vi "rszvl_core_global.vi"() -> ()   [LabVIEW 2014] (continued)
{"Name"="rszvl_rngTrigMode", "Type"=2, "Min?"=FALSE, "Max?"=FALSE, "Entries"=[{"Name"="RSZVL_VAL_TRIG_MODE_IMM", "Discrete or Min"=0.0, "Max"=0.0, "Coerced"=0.0, "Command"="IMM"}, {"Name"="RSZVL_VAL_TRIG_MODE_EXT", "Discrete or Min"=1.0, "Max"=0.0, "Coerced"=0.0, "Command"="EXT"}, {"Name"="RSZVL_VAL_TRIG_MODE_POW", "Discrete or Min"=2.0, "Max"=0.0, "Coerced"=0.0, "Command"="POW"}]}, {"Name"="rszvl_rngWlanDemod", "Type"=2, "Min?"=FALSE, "Max?"=FALSE, "Entries"=[{"Name"="RSZVL_VAL_WLAN_BPSK", "Discrete or Min"=0.0, "Max"=0.0, "Coerced"=0.0, "Command"="BPSK"}, {"Name"="RSZVL_VAL_WLAN_QPSK", "Discrete or Min"=1.0, "Max"=0.0, "Coerced"=0.0, "Command"="QPSK"}, {"Name"="RSZVL_VAL_WLAN_QAM16", "Discrete or Min"=2.0, "Max"=0.0, "Coerced"=0.0, "Command"="QAM16"}, {"Name"="RSZVL_VAL_WLAN_QAM64", "Discrete or Min"=3.0, "Max"=0.0, "Coerced"=0.0, "Command"="QAM64"}, {"Name"="RSZVL_VAL_WLAN_BPSK6", "Discrete or Min"=4.0, "Max"=0.0, "Coerced"=0.0, "Command"="BPSK6"}, {"Name"="RSZVL_VAL_WLAN_BPSK9", "Discrete or Min"=5.0, "Max"=0.0, "Coerced"=0.0, "Command"="BPSK9"}, {"Name"="RSZVL_VAL_WLAN_QPSK12", "Discrete or Min"=6.0, "Max"=0.0, "Coerced"=0.0, "Command"="QPSK12"}, {"Name"="RSZVL_VAL_WLAN_QPSK18", "Discrete or Min"=7.0, "Max"=0.0, "Coerced"=0.0, "Command"="QPSK18"}, {"Name"="RSZVL_VAL_WLAN_QAM1624", "Discrete or Min"=8.0, "Max"=0.0, "Coerced"=0.0, "Command"="QAM1624"}, {"Name"="RSZVL_VAL_WLAN_QAM1636", "Discrete or Min"=9.0, "Max"=0.0, "Coerced"=0.0, "Command"="QAM1636"}, {"Name"="RSZVL_VAL_WLAN_QAM6448", "Discrete or Min"=10.0, "Max"=0.0, "Coerced"=0.0, "Command"="QAM6448"}, {"Name"="RSZVL_VAL_WLAN_QAM6454", "Discrete or Min"=11.0, "Max"=0.0, "Coerced"=0.0, "Command"="QAM6454"}, {"Name"="RSZVL_VAL_WLAN_DBPSK", "Discrete or Min"=12.0, "Max"=0.0, "Coerced"=0.0, "Command"="DBPSK1"}, {"Name"="RSZVL_VAL_WLAN_DQPSK", "Discrete or Min"=13.0, "Max"=0.0, "Coerced"=0.0, "Command"="DQPSK2"}, {"Name"="RSZVL_VAL_WLAN_CCK55", "Discrete or Min"=14.0, "Max"=0.0, "Coerced"=0.0, "Command"="CCK55"}, {"Name"="RSZVL_VAL_WLAN_CCK11", "Discrete or Min"=15.0, "Max"=0.0, "Coerced"=0.0, "Command"="CCK11"}, {"Name"="RSZVL_VAL_WLAN_PBCC55", "Discrete or Min"=16.0, "Max"=0.0, "Coerced"=0.0, "Command"="PBCC55"}, {"Name"="RSZVL_VAL_WLAN_PBCC11", "Discrete or Min"=17.0, "Max"=0.0, "Coerced"=0.0, "Command"="PBCC11"}, {"Name"="RSZVL_VAL_WLAN_PBCC22", "Discrete or Min"=18.0, "Max"=0.0, "Coerced"=0.0, "Command"="PBCC22"}, {"Name"="RSZVL_VAL_WLAN_BPSK3", "Discrete or Min"=19.0, "Max"=0.0, "Coerced"=0.0, "Command"="BPSK3"}, {"Name"="RSZVL_VAL_WLAN_BPSK45", "Discrete or Min"=20.0, "Max"=0.0, "Coerced"=0.0, "Command"="BPSK45"}, {"Name"="RSZVL_VAL_WLAN_QPSK6", "Discrete or Min"=21.0, "Max"=0.0, "Coerced"=0.0, "Command"="QPSK6"}, {"Name"="RSZVL_VAL_WLAN_QPSK9", "Discrete or Min"=22.0, "Max"=0.0, "Coerced"=0.0, "Command"="QPSK9"}, {"Name"="RSZVL_VAL_WLAN_QAM1612", "Discrete or Min"=23.0, "Max"=0.0, "Coerced"=0.0, "Command"="QAM1612"}, {"Name"="RSZVL_VAL_WLAN_QAM1618", "Discrete or Min"=24.0, "Max"=0.0, "Coerced"=0.0, "Command"="QAM1618"}, {"Name"="RSZVL_VAL_WLAN_QAM6424", "Discrete or Min"=25.0, "Max"=0.0, "Coerced"=0.0, "Command"="QAM6424"}, {"Name"="RSZVL_VAL_WLAN_QAM6427", "Discrete or Min"=26.0, "Max"=0.0, "Coerced"=0.0, "Command"="QAM6427"}]}, {"Name"="rszvl_rngWlanDbyte", "Type"=0, "Min?"=TRUE, "Max?"=TRUE, "Entries"=[{"Name"="", "Discrete or Min"=1.0, "Max"=4095.0, "Coerced"=0.0, "Command"=""}]}, {"Name"="rszvl_rngWiMaxStandard", "Type"=0, "Min?"=TRUE, "Max?"=TRUE, "Entries"=[{"Name"="", "Discrete or Min"=0.0, "Max"=2.0, "Coerced"=0.0, "Command"=""}]}, {"Name"="rszvl_rngWiMAXFreqBand", "Type"=2, "Min?"=FALSE, "Max?"=FALSE, "Entries"=[{"Name"="RSZVL_VAL_WIMAX_FBAN_UNSP", "Discrete or Min"=0.0, "Max"=0.0, "Coerced"=0.0, "Command"="UNSP"}, {"Name"="RSZVL_VAL_WIMAX_FBAN_ETSI", "Discrete or Min"=1.0, "Max"=0.0, "Coerced"=0.0, "Command"="ETSI"}, {"Name"="RSZVL_VAL_WIMAX_FBAN_MMDS", "Discrete or Min"=2.0, "Max"=0.0, "Coerced"=0.0, "Command"="MMDS"}, {"Name"="RSZVL_VAL_WIMAX_FBAN_WCS", "Discrete or Min"=3.0, "Max"=0.0, "Coerced"=0.0, "Command"="WCS"}, {"Name"="RSZVL_VAL_WIMAX_FBAN_CEPT", "Discrete or Min"=4.0, "Max"=0.0, "Coerced"=0.0, "Command"="CEPT"}, {"Name"="RSZVL_VAL_WIMAX_FBAN_UNI", "Discrete or Min"=5.0, "Max"=0.0, "Coerced"=0.0, "Command"="UNII"}, {"Name"="RSZVL_VAL_WIMAX_FBAN_ETSI2", "Discrete or Min"=6.0, "Max"=0.0, "Coerced"=0.0, "Command"="ETSI2"}, {"Name"="RSZVL_VAL_WIMAX_FBAN_MMDS2", "Discrete or Min"=7.0, "Max"=0.0, "Coerced"=0.0, "Command"="MMDS2"}, {"Name"="RSZVL_VAL_WIMAX_FBAN_WCS2", "Discrete or Min"=8.0, "Max"=0.0, "Coerced"=0.0, "Command"="WCS2"}, {"Name"="RSZVL_VAL_WIMAX_FBAN_CEPT2", "Discrete or Min"=9.0, "Max"=0.0, "Coerced"=0.0, "Command"="CEPT2"}, {"Name"="RSZVL_VAL_WIMAX_FBAN_UNI2", "Discrete or Min"=10.0, "Max"=0.0, "Coerced"=0.0, "Command"="UNII2"}]}, {"Name"="rszvl_rngWiMAXGuardRatio", "Type"=1, "Min?"=FALSE, "Max?"=FALSE, "Entries"=[{"Name"="", "Discrete or Min"=0.0, "Max"=0.0, "Coerced"=4.0, "Command"=""}, {"Name"="", "Discrete or Min"=0.0, "Max"=0.0, "Coerced"=8.0, "Command"=""}, {"Name"="", "Discrete or Min"=0.0, "Max"=0.0, "Coerced"=16.0, "Command"=""}, {"Name"="", "Discrete or Min"=0.0, "Max"=0.0, "Coerced"=32.0, "Command"=""}]}, {"Name"="rszvl_rngWiMAXRSSIAver", "Type"=0, "Min?"=TRUE, "Max?"=TRUE, "Entries"=[{"Name"="", "Discrete or Min"=1e-06, "Max"=0.999999, "Coerced"=0.0, "Command"=""}]}, {"Name"="rszvl_rngWiMAXModulForm", "Type"=2, "Min?"=FALSE, "Max?"=FALSE, "Entries"=[{"Name"="RSZVL_VAL_WIMAX_MODUL_ALL", "Discrete or Min"=0.0, "Max"=0.0, "Coerced"=0.0, "Command"="ALL"}, {"Name"="RSZVL_VAL_WIMAX_MODUL_QPSK", "Discrete or Min"=1.0, "Max"=0.0, "Coerced"=0.0, "Command"="QPSK"}, {"Name"="RSZVL_VAL_WIMAX_MODUL_QAM16", "Discrete or Min"=2.0, "Max"=0.0, "Coerced"=0.0, "Command"="QAM16"}, {"Name"="RSZVL_VAL_WIMAX_MODUL_QAM64", "Discrete or Min"=3.0, "Max"=0.0, "Coerced"=0.0, "Command"="QAM64"}, {"Name"="RSZVL_VAL_WIMAX_MODUL_BPSK", "Discrete or Min"=4.0, "Max"=0.0, "Coerced"=0.0, "Command"="BPSK"}]}, {"Name"="rszvl_rngWiMAXBurstNumber", "Type"=0, "Min?"=TRUE, "Max?"=TRUE, "Entries"=[{"Name"="", "Discrete or Min"=0.0, "Max"=9999.0, "Coerced"=0.0, "Command"=""}]}, {"Name"="rszvl_rngWiMAXPvtSel", "Type"=2, "Min?"=FALSE, "Max?"=FALSE, "Entries"=[{"Name"="RSZVL_VAL_PVT_EDGE", "Discrete or Min"=0.0, "Max"=0.0, "Coerced"=0.0, "Command"="EDGE"}, {"Name"="RSZVL_VAL_PVT_FULL", "Discrete or Min"=1.0, "Max"=0.0, "Coerced"=0.0, "Command"="FULL"}]}, {"Name"="rszvl_rngHzDeg", "Type"=2, "Min?"=FALSE, "Max?"=FALSE, "Entries"=[{"Name"="RSZVL_VAL_UNIT_DEG", "Discrete or Min"=9.0, "Max"=0.0, "Coerced"=0.0, "Command"="DEG"}, {"Name"="RSZVL_VAL_UNIT_HZ", "Discrete or Min"=12.0, "Max"=0.0, "Coerced"=0.0, "Command"="HZ"}]}, {"Name"="rszvl_rngWiMAXAcpChanNum", "Type"=0, "Min?"=TRUE, "Max?"=TRUE, "Entries"=[{"Name"="", "Discrete or Min"=0.0, "Max"=12.0, "Coerced"=0.0, "Command"=""}]}, {"Name"="rszvl_rngWiMAXChannelBw", "Type"=0, "Min?"=TRUE, "Max?"=TRUE, "Entries"=[{"Name"="", "Discrete or Min"=0.0, "Max"=100000000000.0, "Coerced"=0.0, "Command"=""}]}, {"Name"="rszvl_rngWiMAXChannelSpacing", "Type"=0, "Min?"=TRUE, "Max?"=TRUE, "Entries"=[{"Name"="", "Discrete or Min"=0.0, "Max"=100000000000.0, "Coerced"=0.0, "Command"=""}]}, {"Name"="rszvl_rngWiMAXFlatSel", "Type"=2, "Min?"=FALSE, "Max?"=FALSE, "Entries"=[{"Name"="RSZVL_VAL_WIMAX_FLAT_FLAT", "Discrete or Min"=0.0, "Max"=0.0, "Coerced"=0.0, "Command"="FLAT"}, {"Name"="RSZVL_VAL_WIMAX_FLAT_GRD", "Discrete or Min"=1.0, "Max"=0.0, "Coerced"=0.0, "Command"="GRD"}, {"Name"="RSZVL_VAL_WIMAX_FLAT_DIF", "Discrete or Min"=2.0, "Max"=0.0, "Coerced"=0.0, "Command"="DIFF"}]}, {"Name"="rszvl_rngWiMAXACPRSweepTime", "Type"=0, "Min?"=TRUE, "Max?"=TRUE, "Entries"=[{"Name"="", "Discrete or Min"=0.015, "Max"=16000.0, "Coerced"=0.0, "Command"=""}]}, {"Name"="rszvl_rngWiMAXDemod", "Type"=2, "Min?"=FALSE, "Max?"=FALSE, "Entries"=[{"Name"="RSZVL_VAL_WIMAX_BPSK1_2", "Discrete or Min"=0.0, "Max"=0.0, "Coerced"=0.0, "Command"="BPSK1/2"}, {"Name"="RSZVL_VAL_WIMAX_QPSK1_2", "Discrete or Min"=1.0, "Max"=0.0, "Coerced"=0.0, "Command"="QPSK1/2"}, {"Name"="RSZVL_VAL_WIMAX_QPSK3_4", "Discrete or Min"=2.0, "Max"=0.0, "Coerced"=0.0, "Command"="QPSK3/4"}, {"Name"="RSZVL_VAL_WIMAX_16QAM1_2", "Discrete or Min"=3.0, "Max"=0.0, "Coerced"=0.0, "Command"="16QAM1/2"}, {"Name"="RSZVL_VAL_WIMAX_16QAM3_4", "Discrete or Min"=4.0, "Max"=0.0, "Coerced"=0.0, "Command"="16QAM3/4"}, {"Name"="RSZVL_VAL_WIMAX_64QAM2_3", "Discrete or Min"=5.0, "Max"=0.0, "Coerced"=0.0, "Command"="64QAM2/3"}, {"Name"="RSZVL_VAL_WIMAX_64QAM3_4", "Discrete or Min"=6.0, "Max"=0.0, "Coerced"=0.0, "Command"="64QAM3/4"}]}, {"Name"="rszvl_rngWiMAXBconAuto", "Type"=2, "Min?"=FALSE, "Max?"=FALSE, "Entries"=[{"Name"="RSZVL_VAL_WIMAX_BCON_NONE", "Discrete or Min"=0.0, "Max"=0.0, "Coerced"=0.0, "Command"="NONE"}, {"Name"="RSZVL_VAL_WIMAX_BCON_FIRST", "Discrete or Min"=1.0, "Max"=0.0, "Coerced"=0.0, "Command"="FIRS"}, {"Name"="RSZVL_VAL_WIMAX_BCON_USER", "Discrete or Min"=2.0, "Max"=0.0, "Coerced"=0.0, "Command"="USER"}, {"Name"="RSZVL_VAL_WIMAX_BCON_ALL", "Discrete or Min"=3.0, "Max"=0.0, "Coerced"=0.0, "Command"="ALL"}, {"Name"="RSZVL_VAL_WIMAX_BCON_SIGNAL", "Discrete or Min"=4.0, "Max"=0.0, "Coerced"=0.0, "Command"="SIGN"}, {"Name"="RSZVL_VAL_WIMAX_BCON_PREDEF", "Discrete or Min"=5.0, "Max"=0.0, "Coerced"=0.0, "Command"="PRED"}]}, {"Name"="rszvl_rngWiMAXLinkMode", "Type"=2, "Min?"=FALSE, "Max?"=FALSE, "Entries"=[{"Name"="RSZVL_VAL_WIMAX_LMOD_DL", "Discrete or Min"=0.0, "Max"=0.0, "Coerced"=0.0, "Command"="DL"}, {"Name"="RSZVL_VAL_WIMAX_LMOD_UL", "Discrete or Min"=1.0, "Max"=0.0, "Coerced"=0.0, "Command"="UL"}]}, {"Name"="rszvl_rngSubchannel", "Type"=0, "Min?"=TRUE, "Max?"=TRUE, "Entries"=[{"Name"="", "Discrete or Min"=1.0, "Max"=31.0, "Coerced"=0.0, "Command"=""}]}, {"Name"="rszvl_rngSubchannelULPH", "Type"=0, "Min?"=TRUE, "Max?"=TRUE, "Entries"=[{"Name"="", "Discrete or Min"=0.0, "Max"=255.0, "Coerced"=0.0, "Command"=""}]}, {"Name"="rszvl_rngWiMAXCestType", "Type"=2, "Min?"=FALSE, "Max?"=FALSE, "Entries"=[{"Name"="RSZVL_VAL_WIMAX_CEST_PREAMONLY", "Discrete or Min"=0.0, "Max"=0.0, "Coerced"=0.0, "Command"="PREamonly"}, {"Name"="RSZVL_VAL_WIMAX_CEST_PREAMPAYL", "Discrete or Min"=1.0, "Max"=0.0, "Coerced"=0.0, "Command"="PREampayl"}, {"Name"="RSZVL_VAL_WIMAX_CEST_PAYLONLY", "Discrete or Min"=2.0, "Max"=0.0, "Coerced"=0.0, "Command"="PAYLonly"}]}, {"Name"="rszvl_rngWiMAXTracPilots", "Type"=2, "Min?"=FALSE, "Max?"=FALSE, "Entries"=[{"Name"="RSZVL_VAL_WIMAX_TRAC_PIL_PRED", "Discrete or Min"=0.0, "Max"=0.0, "Coerced"=0.0, "Command"="PRED"}, {"Name"="RSZVL_VAL_WIMAX_TRAC_PIL_DET", "Discrete or Min"=1.0, "Max"=0.0, "Coerced"=0.0, "Command"="DET"}]}, {"Name"="rszvl_rngWiMAXDLFramePreMode", "Type"=2, "Min?"=FALSE, "Max?"=FALSE, "Entries"=[{"Name"="RSZVL_VAL_WIMAX_PRE_AUTO", "Discrete or Min"=0.0, "Max"=0.0, "Coerced"=0.0, "Command"="AUTO"}, {"Name"="RSZVL_VAL_WIMAX_PRE_USER", "Discrete or Min"=1.0, "Max"=0.0, "Coerced"=0.0, "Command"="USER"}]}, {"Name"="rszvl_rngWiMAXDLFramePreIndex", "Type"=0, "Min?"=TRUE, "Max?"=TRUE, "Entries"=[{"Name"="", "Discrete or Min"=0.0, "Max"=113.0, "Coerced"=0.0, "Command"=""}]}, {"Name"="rszvl_rngWiMAXZoneType", "Type"=2, "Min?"=FALSE, "Max?"=FALSE, "Entries"=[{"Name"="RSZVL_VAL_WIMAX_ZONE_TYPE_DLFUSC", "Discrete or Min"=0.0, "Max"=0.0, "Coerced"=0.0, "Command"="DLFUSC"}, {"Name"="RSZVL_VAL_WIMAX_ZONE_TYPE_DLPUSC", "Discrete or Min"=1.0, "Max"=0.0, "Coerced"=0.0, "Command"="DLPUSC"}, {"Name"="RSZVL_VAL_WIMAX_ZONE_TYPE_ULPUSC", "Discrete or Min"=2.0, "Max"=0.0, "Coerced"=0.0, "Command"="ULPUSC"}]}, {"Name"="rszvl_rngWiMAXZoneSegNum", "Type"=0, "Min?"=TRUE, "Max?"=TRUE, "Entries"=[{"Name"="", "Discrete or Min"=0.0, "Max"=2.0, "Coerced"=0.0, "Command"=""}]}, {"Name"="rszvl_rngWiMAXZoneBurstFormat", "Type"=2, "Min?"=FALSE, "Max?"=FALSE, "Entries"=[{"Name"="RSZVL_VAL_WIMAX_ZONE_BURST_FORM_QPSK_12", "Discrete or Min"=0.0, "Max"=0.0, "Coerced"=0.0, "Command"="QPSK_1_2"}, {"Name"="RSZVL_VAL_WIMAX_ZONE_BURST_FORM_QPSK_34", "Discrete or Min"=1.0, "Max"=0.0, "Coerced"=0.0, "Command"="QPSK_3_4"}, {"Name"="RSZVL_VAL_WIMAX_ZONE_BURST_FORM_QAM16_12", "Discrete or Min"=2.0, "Max"=0.0, "Coerced"=0.0, "Command"="QAM16_1_2"}, {"Name"="RSZVL_VAL_WIMAX_ZONE_BURST_FORM_QAM16_34", "Discrete or Min"=3.0, "Max"=0.0, "Coerced"=0.0, "Command"="QAM16_3_4"}, {"Name"="RSZVL_VAL_WIMAX_ZONE_BURST_FORM_QAM64_12", "Discrete or Min"=4.0, "Max"=0.0, "Coerced"=0.0, "Command"="QAM64_1_2"}, {"Name"="RSZVL_VAL_WIMAX_ZONE_BURST_FORM_QAM64_23", "Discrete or Min"=5.0, "Max"=0.0, "Coerced"=0.0, "Command"="QAM64_2_3"}, {"Name"="RSZVL_VAL_WIMAX_ZONE_BURST_FORM_QAM64_34", "Discrete or Min"=6.0, "Max"=0.0, "Coerced"=0.0, "Command"="QAM64_3_4"}]}, {"Name"="rszvl_rngWiMAXZoneBurstSlotDuration", "Type"=0, "Min?"=TRUE, "Max?"=TRUE, "Entries"=[{"Name"="", "Discrete or Min"=0.0, "Max"=3000.0, "Coerced"=0.0, "Command"=""}]}, {"Name"="rszvl_rngWiMAXZoneBurstSChanCount", "Type"=0, "Min?"=TRUE, "Max?"=TRUE, "Entries"=[{"Name"="", "Discrete or Min"=1.0, "Max"=30.0, "Coerced"=0.0, "Command"=""}]}, {"Name"="rszvl_rngWiMAXZoneBurstSymbCount", "Type"=0, "Min?"=TRUE, "Max?"=TRUE, "Entries"=[{"Name"="", "Discrete or Min"=2.0, "Max"=1000.0, "Coerced"=0.0, "Command"=""}]}, {"Name"="rszvl_rngWiMAXZoneBurstSymbOffset", "Type"=0, "Min?"=TRUE, "Max?"=TRUE, "Entries"=[{"Name"="", "Discrete or Min"=0.0, "Max"=1000.0, "Coerced"=0.0, "Command"=""}]}, {"Name"="rszvl_rngWiMAXZoneBurstType", "Type"=2, "Min?"=FALSE, "Max?"=FALSE, "Entries"=[{"Name"="RSZVL_VAL_WIMAX_ZONE_BURS_TYPE_FCH", "Discrete or Min"=0.0, "Max"=0.0, "Coerced"=0.0, "Command"="FCH"}, {"Name"="RSZVL_VAL_WIMAX_ZONE_BURS_TYPE_DLMAP", "Discrete or Min"=1.0, "Max"=0.0, "Coerced"=0.0, "Command"="DLMAP"}, {"Name"="RSZVL_VAL_WIMAX_ZONE_BURS_TYPE_ULMAP", "Discrete or Min"=2.0, "Max"=0.0, "Coerced"=0.0, "Command"="ULMAP"}, {"Name"="RSZVL_VAL_WIMAX_ZONE_BURS_TYPE_DATA", "Discrete or Min"=3.0, "Max"=0.0, "Coerced"=0.0, "Command"="DATA"}]}, {"Name"="rszvl_rngTriggerSourceB6", "Type"=2, "Min?"=FALSE, "Max?"=FALSE, "Entries"=[{"Name"="RSZVL_VAL_TRG_B6_TV", "Discrete or Min"=0.0, "Max"=0.0, "Coerced"=0.0, "Command"="TV"}]}, {"Name"="rszvl_rngTriggerTVVertSig", "Type"=2, "Min?"=FALSE, "Max?"=FALSE, "Entries"=[{"Name"="RSZVL_VAL_TRIG_TV_VFIEL_ALL", "Discrete or Min"=0.0, "Max"=0.0, "Coerced"=0.0, "Command"="ALL"}, {"Name"="RSZVL_VAL_TRIG_TV_VFIEL_ODD", "Discrete or Min"=1.0, "Max"=0.0, "Coerced"=0.0, "Command"="ODD"}, {"Name"="RSZVL_VAL_TRIG_TV_VFIEL_EVEN", "Discrete or Min"=2.0, "Max"=0.0, "Coerced"=0.0, "Command"="EVEN"}, {"Name"="RSZVL_VAL_TRIG_TV_HORIZONTAL", "Discrete or Min"=3.0, "Max"=0.0, "Coerced"=0.0, "Command"="HOR"}]}, {"Name"="rszvl_rngTriggerTVLineSystem", "Type"=1, "Min?"=FALSE, "Max?"=FALSE, "Entries"=[{"Name"="", "Discrete or Min"=0.0, "Max"=0.0, "Coerced"=525.0, "Command"=""}, {"Name"="", "Discrete or Min"=0.0, "Max"=0.0, "Coerced"=625.0, "Command"=""}]}, {"Name"="rszvl_rngDISPFormat", "Type"=2, "Min?"=FALSE, "Max?"=FALSE, "Entries"=[{"Name"="RSZVL_VAL_DISP_FORMAT_SINGLE", "Discrete or Min"=0.0, "Max"=0.0, "Coerced"=0.0, "Command"="SING"}, {"Name"="RSZVL_VAL_DISP_FORMAT_SPLIT", "Discrete or Min"=1.0, "Max"=0.0, "Coerced"=0.0, "Command"="SPL"}]}, {"Name"="rszvl_rngBtoChannel", "Type"=0, "Min?"=TRUE, "Max?"=TRUE, "Entries"=[{"Name"="", "Discrete or Min"=0.0, "Max"=78.0, "Coerced"=0.0, "Command"=""}]}, {"Name"="rszvl_rngIQSRateB72", "Type"=0, "Min?"=TRUE, "Max?"=TRUE, "Entries"=[{"Name"="", "Discrete or Min"=41667.0, "Max"=326400000.0, "Coerced"=0.0, "Command"=""}]}, {"Name"="rszvl_rngSpemAnalysis", "Type"=2, "Min?"=FALSE, "Max?"=FALSE, "Entries"=[{"Name"="RSZVL_VAL_SPEM_ANALYSIS_DL", "Discrete or Min"=0.0, "Max"=0.0, "Coerced"=0.0, "Command"="DL"}, {"Name"="RSZVL_VAL_SPEM_ANALYSIS_UL", "Discrete or Min"=1.0, "Max"=0.0, "Coerced"=0.0, "Command"="UL"}]}, {"Name"="rszvl_rngWiMAXExtTrgLev", "Type"=0, "Min?"=TRUE, "Max?"=TRUE, "Entries"=[{"Name"="", "Discrete or Min"=0.5, "Max"=3.5, "Coerced"=0.0, "Command"=""}]}, {"Name"="rszvl_rngWiMAXSignalInput", "Type"=2, "Min?"=FALSE, "Max?"=FALSE, "Entries"=[{"Name"="RSZVL_VAL_WIMAX_SIGNAL_INP_RF", "Discrete or Min"=0.0, "Max"=0.0, "Coerced"=0.0, "Command"="RF"}]}, {"Name"="rszvl_rngWiMAXESPTTA", "Type"=2, "Min?"=FALSE, "Max?"=FALSE, "Entries"=[{"Name"="RSZVL_VAL_WIMAX_ESP_TTA_STAN", "Discrete or Min"=0.0, "Max"=0.0, "Coerced"=0.0, "Command"="STAN"}, {"Name"="RSZVL_VAL_WIMAX_ESP_TTA_USER", "Discrete or Min"=1.0, "Max"=0.0, "Coerced"=0.0, "Command"="USER"}]}, {"Name"="rszvl_rng3GPPESPMode", "Type"=2, "Min?"=FALSE, "Max?"=FALSE, "Entries"=[{"Name"="RSZVL_VAL_3GPP_ESP_MODE_AUTO", "Discrete or Min"=0.0, "Max"=0.0, "Coerced"=0.0, "Command"="AUTO"}, {"Name"="RSZVL_VAL_3GPP_ESP_MODE_MAN", "Discrete or Min"=1.0, "Max"=0.0, "Coerced"=0.0, "Command"="MAN"}, {"Name"="RSZVL_VAL_3GPP_ESP_MODE_USER", "Discrete or Min"=2.0, "Max"=0.0, "Coerced"=0.0, "Command"="USER"}]}, {"Name"="rszvl_rng3GPESPTransition", "Type"=0, "Min?"=TRUE, "Max?"=TRUE, "Entries"=[{"Name"="", "Discrete or Min"=100.0, "Max"=1000000000.0, "Coerced"=0.0, "Command"=""}]}, {"Name"="rszvl_rng3GPPESPPredefinedLimLine", "Type"=1, "Min?"=FALSE, "Max?"=FALSE, "Entries"=[{"Name"="", "Discrete or Min"=0.0, "Max"=0.0, "Coerced"=0.0, "Command"=""}, {"Name"="", "Discrete or Min"=0.0, "Max"=0.0, "Coerced"=31.0, "Command"=""}, {"Name"="", "Discrete or Min"=0.0, "Max"=0.0, "Coerced"=39.0, "Command"=""}, {"Name"="", "Discrete or Min"=0.0, "Max"=0.0, "Coerced"=43.0, "Command"=""}]}, {"Name"="rszvl_rngNoiseMarkerTrace", "Type"=2, "Min?"=FALSE, "Max?"=FALSE, "Entries"=[{"Name"="RSZVL_VAL_NOISE_MARKER_TRACE_NOIS", "Discrete or Min"=0.0, "Max"=0.0, "Coerced"=0.0, "Command"="NOIS"}, {"Name"="RSZVL_VAL_NOISE_MARKER_TRACE_GAIN", "Discrete or Min"=1.0, "Max"=0.0, "Coerced"=0.0, "Command"="GAIN"}]}, {"Name"="rszvl_rngCatvFreqOffset", "Type"=0, "Min?"=TRUE, "Max?"=TRUE, "Entries"=[{"Name"="", "Discrete or Min"=-999999.0, "Max"=999999.0, "Coerced"=0.0, "Command"=""}]}, {"Name"="rszvl_rngCatvRelPower", "Type"=0, "Min?"=TRUE, "Max?"=TRUE, "Entries"=[{"Name"="", "Discrete or Min"=-200.0, "Max"=200.0, "Coerced"=0.0, "Command"=""}]}, {"Name"="rszvl_rngCatvAbsPower", "Type"=0, "Min?"=TRUE, "Max?"=TRUE, "Entries"=[{"Name"="", "Discrete or Min"=-200.0, "Max"=200.0, "Coerced"=0.0, "Command"=""}]}, {"Name"="rszvl_rngCatvHumLimitUpper", "Type"=0, "Min?"=TRUE, "Max?"=TRUE, "Entries"=[{"Name"="", "Discrete or Min"=0.1, "Max"=100.0, "Coerced"=0.0, "Command"=""}]}, {"Name"="rszvl_rngCatvHumLimitLower", "Type"=0, "Min?"=TRUE, "Max?"=TRUE, "Entries"=[{"Name"="", "Discrete or Min"=-60.0, "Max"=60.0, "Coerced"=0.0, "Command"=""}]}, {"Name"="rszvl_rngCatvCarrSuppression", "Type"=0, "Min?"=TRUE, "Max?"=TRUE, "Entries"=[{"Name"="", "Discrete or Min"=0.0, "Max"=200.0, "Coerced"=0.0, "Command"=""}]}, {"Name"="rszvl_rngCatvErrLimitLower", "Type"=0, "Min?"=TRUE, "Max?"=TRUE, "Entries"=[{"Name"="", "Discrete or Min"=0.0, "Max"=80.0, "Coerced"=0.0, "Command"=""}]}, {"Name"="rszvl_rngCatvErrLimitUpper", "Type"=0, "Min?"=TRUE, "Max?"=TRUE, "Entries"=[{"Name"="", "Discrete or Min"=0.01, "Max"=100.0, "Coerced"=0.0, "Command"=""}]}, {"Name"="rszvl_rngCatvImbLimit", "Type"=0, "Min?"=TRUE, "Max?"=TRUE, "Entries"=[{"Name"="", "Discrete or Min"=-100.0, "Max"=100.0, "Coerced"=0.0, "Command"=""}]}, {"Name"="rszvl_rngCatvPhaseJitterLimit", "Type"=0, "Min?"=TRUE, "Max?"=TRUE, "Entries"=[{"Name"="", "Discrete or Min"=0.0, "Max"=180.0, "Coerced"=0.0, "Command"=""}]}, {"Name"="rszvl_rngCatvQuadratureErrLimit", "Type"=0, "Min?"=TRUE, "Max?"=TRUE, "Entries"=[{"Name"="", "Discrete or Min"=-180.0, "Max"=180.0, "Coerced"=0.0, "Command"=""}]}, {"Name"="rszvl_rngCatvSymbRateLimit", "Type"=0, "Min?"=TRUE, "Max?"=TRUE, "Entries"=[{"Name"="", "Discrete or Min"=-99999.0, "Max"=99999.0, "Coerced"=0.0, "Command"=""}]}, {"Name"="rszvl_rngUnitSecMin", "Type"=2, "Min?"=FALSE, "Max?"=FALSE, "Entries"=[{"Name"="RSZVL_VAL_UNIT_SEC", "Discrete or Min"=0.0, "Max"=0.0, "Coerced"=0.0, "Command"="s"}, {"Name"="RSZVL_VAL_UNIT_MIN", "Discrete or Min"=1.0, "Max"=0.0, "Coerced"=0.0, "Command"="m"}]}, {"Name"="rszvl_rngCatvAtvCarrMeas", "Type"=2, "Min?"=FALSE, "Max?"=FALSE, "Entries"=[{"Name"="RSZVL_VAL_ATV_MEAS_CARR_CARR", "Discrete or Min"=0.0, "Max"=0.0, "Coerced"=0.0, "Command"="CARR"}, {"Name"="RSZVL_VAL_ATV_MEAS_CARR_NOIS", "Discrete or Min"=1.0, "Max"=0.0, "Coerced"=0.0, "Command"="NOIS"}]}, {"Name"="rszvl_rngCatvAtvMeas", "Type"=2, "Min?"=FALSE, "Max?"=FALSE, "Entries"=[{"Name"="RSZVL_VAL_ATV_MEAS_ASP", "Discrete or Min"=0.0, "Max"=0.0, "Coerced"=0.0, "Command"="ASP"}, {"Name"="RSZVL_VAL_ATV_MEAS_CARR", "Discrete or Min"=1.0, "Max"=0.0, "Coerced"=0.0, "Command"="CARR"}, {"Name"="RSZVL_VAL_ATV_MEAS_CN", "Discrete or Min"=2.0, "Max"=0.0, "Coerced"=0.0, "Command"="CN"}, {"Name"="RSZVL_VAL_ATV_MEAS_CSO", "Discrete or Min"=3.0, "Max"=0.0, "Coerced"=0.0, "Command"="CSO"}, {"Name"="RSZVL_VAL_ATV_MEAS_CTB", "Discrete or Min"=4.0, "Max"=0.0, "Coerced"=0.0, "Command"="CTB"}, {"Name"="RSZVL_VAL_ATV_MEAS_HUM", "Discrete or Min"=5.0, "Max"=0.0, "Coerced"=0.0, "Command"="HUM"}, {"Name"="RSZVL_VAL_ATV_MEAS_VMOD", "Discrete or Min"=6.0, "Max"=0.0, "Coerced"=0.0, "Command"="VMOD"}, {"Name"="RSZVL_VAL_ATV_MEAS_VSC", "Discrete or Min"=7.0, "Max"=0.0, "Coerced"=0.0, "Command"="VSC"}]}, {"Name"="rszvl_rngCatvDtvMeas", "Type"=2, "Min?"=FALSE, "Max?"=FALSE, "Entries"=[{"Name"="RSZVL_VAL_DTV_MEAS_DSP", "Discrete or Min"=0.0, "Max"=0.0, "Coerced"=0.0, "Command"="DSP"}, {"Name"="RSZVL_VAL_DTV_MEAS_CHP", "Discrete or Min"=1.0, "Max"=0.0, "Coerced"=0.0, "Command"="CHP"}, {"Name"="RSZVL_VAL_DTV_MEAS_CONS", "Discrete or Min"=2.0, "Max"=0.0, "Coerced"=0.0, "Command"="CONS"}, {"Name"="RSZVL_VAL_DTV_MEAS_MERR", "Discrete or Min"=3.0, "Max"=0.0, "Coerced"=0.0, "Command"="MERR"}, {"Name"="RSZVL_VAL_DTV_MEAS_EPATT", "Discrete or Min"=4.0, "Max"=0.0, "Coerced"=0.0, "Command"="EPAT"}, {"Name"="RSZVL_VAL_DTV_MEAS_APD", "Discrete or Min"=5.0, "Max"=0.0, "Coerced"=0.0, "Command"="APD"}, {"Name"="RSZVL_VAL_DTV_MEAS_CCDF", "Discrete or Min"=6.0, "Max"=0.0, "Coerced"=0.0, "Command"="CCDF"}, {"Name"="RSZVL_VAL_DTV_MEAS_OVER", "Discrete or Min"=7.0, "Max"=0.0, "Coerced"=0.0, "Command"="OVER"}]}, {"Name"="rszvl_rngCatvTvMeas", "Type"=2, "Min?"=FALSE, "Max?"=FALSE, "Entries"=[{"Name"="RSZVL_VAL_TV_MEAS_TILT", "Discrete or Min"=0.0, "Max"=0.0, "Coerced"=0.0, "Command"="TILT"}]}, {"Name"="rszvl_rngCatvEpattZoom", "Type"=0, "Min?"=TRUE, "Max?"=TRUE, "Entries"=[{"Name"="", "Discrete or Min"=1.0, "Max"=20.0, "Coerced"=0.0, "Command"=""}]}, {"Name"="rszvl_rngCatvMerrZoom", "Type"=2, "Min?"=FALSE, "Max?"=FALSE, "Entries"=[{"Name"="RSZVL_VAL_CATV_MERR_ZOOM_NONE", "Discrete or Min"=0.0, "Max"=0.0, "Coerced"=0.0, "Command"="NONE"}, {"Name"="RSZVL_VAL_CATV_MERR_ZOOM_MERR", "Discrete or Min"=1.0, "Max"=0.0, "Coerced"=0.0, "Command"="MERR"}, {"Name"="RSZVL_VAL_CATV_MERR_ZOOM_MERP", "Discrete or Min"=2.0, "Max"=0.0, "Coerced"=0.0, "Command"="MERP"}, {"Name"="RSZVL_VAL_CATV_MERR_ZOOM_EVMR", "Discrete or Min"=3.0, "Max"=0.0, "Coerced"=0.0, "Command"="EVMR"}, {"Name"="RSZVL_VAL_CATV_MERR_ZOOM_EVMP", "Discrete or Min"=4.0, "Max"=0.0, "Coerced"=0.0, "Command"="EVMP"}, {"Name"="RSZVL_VAL_CATV_MERR_ZOOM_IMB", "Discrete or Min"=5.0, "Max"=0.0, "Coerced"=0.0, "Command"="IMB"}, {"Name"="RSZVL_VAL_CATV_MERR_ZOOM_QERR", "Discrete or Min"=6.0, "Max"=0.0, "Coerced"=0.0, "Command"="QERR"}, {"Name"="RSZVL_VAL_CATV_MERR_ZOOM_SUP", "Discrete or Min"=7.0, "Max"=0.0, "Coerced"=0.0, "Command"="SUPP"}, {"Name"="RSZVL_VAL_CATV_MERR_ZOOM_PJIT", "Discrete or Min"=8.0, "Max"=0.0, "Coerced"=0.0, "Command"="PJIT"}]}, {"Name"="rszvl_rngCatvOverZoom", "Type"=2, "Min?"=FALSE, "Max?"=FALSE, "Entries"=[{"Name"="RSZVL_VAL_CATV_OVER_ZOOM_NONE", "Discrete or Min"=0.0, "Max"=0.0, "Coerced"=0.0, "Command"="NONE"}, {"Name"="RSZVL_VAL_CATV_OVER_ZOOM_MERR", "Discrete or Min"=1.0, "Max"=0.0, "Coerced"=0.0, "Command"="MERR"}, {"Name"="RSZVL_VAL_CATV_OVER_ZOOM_MERP", "Discrete or Min"=2.0, "Max"=0.0, "Coerced"=0.0, "Command"="MERP"}, {"Name"="RSZVL_VAL_CATV_OVER_ZOOM_EVMR", "Discrete or Min"=3.0, "Max"=0.0, "Coerced"=0.0, "Command"="EVMR"}, {"Name"="RSZVL_VAL_CATV_OVER_ZOOM_EVMP", "Discrete or Min"=4.0, "Max"=0.0, "Coerced"=0.0, "Command"="EVMP"}, {"Name"="RSZVL_VAL_CATV_OVER_ZOOM_CFOF", "Discrete or Min"=5.0, "Max"=0.0, "Coerced"=0.0, "Command"="CFOF"}, {"Name"="RSZVL_VAL_CATV_OVER_ZOOM_SROF", "Discrete or Min"=6.0, "Max"=0.0, "Coerced"=0.0, "Command"="SROF"}]}, {"Name"="rszvl_rngCatvConstDiagZoom", "Type"=2, "Min?"=FALSE, "Max?"=FALSE, "Entries"=[{"Name"="RSZVL_VAL_CATV_QUAD_ZOOM_NONE", "Discrete or Min"=0.0, "Max"=0.0, "Coerced"=0.0, "Command"="NONE"}, {"Name"="RSZVL_VAL_CATV_QUAD_ZOOM_1", "Discrete or Min"=1.0, "Max"=0.0, "Coerced"=0.0, "Command"="1"}, {"Name"="RSZVL_VAL_CATV_QUAD_ZOOM_2", "Discrete or Min"=2.0, "Max"=0.0, "Coerced"=0.0, "Command"="2"}, {"Name"="RSZVL_VAL_CATV_QUAD_ZOOM_3", "Discrete or Min"=3.0, "Max"=0.0, "Coerced"=0.0, "Command"="3"}, {"Name"="RSZVL_VAL_CATV_QUAD_ZOOM_4", "Discrete or Min"=4.0, "Max"=0.0, "Coerced"=0.0, "Command"="4"}]}, {"Name"="rszvl_rngCatvAtvBw", "Type"=0, "Min?"=TRUE, "Max?"=TRUE, "Entries"=[{"Name"="", "Discrete or Min"=100.0, "Max"=20000000.0, "Coerced"=0.0, "Command"=""}]}, {"Name"="rszvl_rngCatvAtvCarrMeasMode", "Type"=2, "Min?"=FALSE, "Max?"=FALSE, "Entries"=[{"Name"="RSZVL_VAL_ATV_MEAS_MODE_INSERVICE", "Discrete or Min"=0.0, "Max"=0.0, "Coerced"=0.0, "Command"="ISER"}, {"Name"="RSZVL_VAL_ATV_MEAS_MODE_OFFSERVICE", "Discrete or Min"=1.0, "Max"=0.0, "Coerced"=0.0, "Command"="OSER"}, {"Name"="RSZVL_VAL_ATV_MEAS_MODE_QUIETLINE", "Discrete or Min"=2.0, "Max"=0.0, "Coerced"=0.0, "Command"="QLIN"}]}, {"Name"="rszvl_rngCatvAtvRefPowerMode", "Type"=2, "Min?"=FALSE, "Max?"=FALSE, "Entries"=[{"Name"="RSZVL_VAL_ATV_RPOW_MODE_RCH", "Discrete or Min"=0.0, "Max"=0.0, "Coerced"=0.0, "Command"="RCH"}, {"Name"="RSZVL_VAL_ATV_RPOW_MODE_MCH", "Discrete or Min"=1.0, "Max"=0.0, "Coerced"=0.0, "Command"="MCH"}, {"Name"="RSZVL_VAL_ATV_RPOW_MODE_MAN", "Discrete or Min"=2.0, "Max"=0.0, "Coerced"=0.0, "Command"="MAN"}]}, {"Name"="rszvl_rngCatvDtvEPattVelocity", "Type"=0, "Min?"=TRUE, "Max?"=TRUE, "Entries"=[{"Name"="", "Discrete or Min"=0.0001, "Max"=1.0, "Coerced"=0.0, "Command"=""}]}, {"Name"="rszvl_rngCatvDtvFilterAlpha", "Type"=2, "Min?"=FALSE, "Max?"=FALSE, "Entries"=[{"Name"="RSZVL_VAL_CATV_DTV_ALPHA_R012", "Discrete or Min"=0.0, "Max"=0.0, "Coerced"=0.0, "Command"="R012"}, {"Name"="RSZVL_VAL_CATV_DTV_ALPHA_R013", "Discrete or Min"=1.0, "Max"=0.0, "Coerced"=0.0, "Command"="R013"}, {"Name"="RSZVL_VAL_CATV_DTV_ALPHA_R015", "Discrete or Min"=2.0, "Max"=0.0, "Coerced"=0.0, "Command"="R015"}, {"Name"="RSZVL_VAL_CATV_DTV_ALPHA_R018", "Discrete or Min"=3.0, "Max"=0.0, "Coerced"=0.0, "Command"="R018"}]}, {"Name"="rszvl_rngCatvSBand", "Type"=2, "Min?"=FALSE, "Max?"=FALSE, "Entries"=[{"Name"="RSZVL_VAL_CATV_SBAND_NORM", "Discrete or Min"=0.0, "Max"=0.0, "Coerced"=0.0, "Command"="NORM"}, {"Name"="RSZVL_VAL_CATV_SBAND_INV", "Discrete or Min"=1.0, "Max"=0.0, "Coerced"=0.0, "Command"="INV"}, {"Name"="RSZVL_VAL_CATV_SBAND_AUTO", "Discrete or Min"=2.0, "Max"=0.0, "Coerced"=0.0, "Command"="AUTO"}]}, {"Name"="rszvl_rngCatvRFFreq", "Type"=0, "Min?"=TRUE, "Max?"=TRUE, "Entries"=[{"Name"="", "Discrete or Min"=5000000.0, "Max"=1000000000.0, "Coerced"=0.0, "Command"=""}]}, {"Name"="rszvl_rngCatvModStandGroupDelay", "Type"=2, "Min?"=FALSE, "Max?"=FALSE, "Entries"=[{"Name"="RSZVL_VAL_CATV_GDELAY_GENERAL", "Discrete or Min"=0.0, "Max"=0.0, "Coerced"=0.0, "Command"="GEN"}, {"Name"="RSZVL_VAL_CATV_GDELAY_GHALF", "Discrete or Min"=1.0, "Max"=0.0, "Coerced"=0.0, "Command"="GHAL"}, {"Name"="RSZVL_VAL_CATV_GDELAY_AUSTRALIA", "Discrete or Min"=2.0, "Max"=0.0, "Coerced"=0.0, "Command"="AUST"}, {"Name"="RSZVL_VAL_CATV_GDELAY_DANMARK", "Discrete or Min"=3.0, "Max"=0.0, "Coerced"=0.0, "Command"="DANM"}, {"Name"="RSZVL_VAL_CATV_GDELAY_NEWZELAND", "Discrete or Min"=4.0, "Max"=0.0, "Coerced"=0.0, "Command"="NEWZ"}, {"Name"="RSZVL_VAL_CATV_GDELAY_NORWAY", "Discrete or Min"=5.0, "Max"=0.0, "Coerced"=0.0, "Command"="NORW"}, {"Name"="RSZVL_VAL_CATV_GDELAY_SWEDENFULL", "Discrete or Min"=6.0, "Max"=0.0, "Coerced"=0.0, "Command"="SWED"}, {"Name"="RSZVL_VAL_CATV_GDELAY_FLAT", "Discrete or Min"=7.0, "Max"=0.0, "Coerced"=0.0, "Command"="FLAT"}, {"Name"="RSZVL_VAL_CATV_GDELAY_OIRT", "Discrete or Min"=8.0, "Max"=0.0, "Coerced"=0.0, "Command"="OIRT"}, {"Name"="RSZVL_VAL_CATV_GDELAY_CHINA", "Discrete or Min"=9.0, "Max"=0.0, "Coerced"=0.0, "Command"="CHIN"}, {"Name"="RSZVL_VAL_CATV_GDELAY_CCIR", "Discrete or Min"=10.0, "Max"=0.0, "Coerced"=0.0, "Command"="CCIR"}, {"Name"="RSZVL_VAL_CATV_GDELAY_TDF", "Discrete or Min"=11.0, "Max"=0.0, "Coerced"=0.0, "Command"="TDF"}, {"Name"="RSZVL_VAL_CATV_GDELAY_FFC", "Discrete or Min"=12.0, "Max"=0.0, "Coerced"=0.0, "Command"="FFC"}]}, {"Name"="rszvl_rngCatvModStandSignalType", "Type"=2, "Min?"=FALSE, "Max?"=FALSE, "Entries"=[{"Name"="RSZVL_VAL_CATV_SIG_TYPE_ATV", "Discrete or Min"=0.0, "Max"=0.0, "Coerced"=0.0, "Command"="ATV"}, {"Name"="RSZVL_VAL_CATV_SIG_TYPE_DTV", "Discrete or Min"=1.0, "Max"=0.0, "Coerced"=0.0, "Command"="DTV"}]}, {"Name"="rszvl_rngCatvAtvStandard", "Type"=2, "Min?"=FALSE, "Max?"=FALSE, "Entries"=[{"Name"="RSZVL_VAL_ATV_STAN_BG", "Discrete or Min"=0.0, "Max"=0.0, "Coerced"=0.0, "Command"="BG"}, {"Name"="RSZVL_VAL_ATV_STAN_DK", "Discrete or Min"=1.0, "Max"=0.0, "Coerced"=0.0, "Command"="DK"}, {"Name"="RSZVL_VAL_ATV_STAN_I", "Discrete or Min"=2.0, "Max"=0.0, "Coerced"=0.0, "Command"="I"}, {"Name"="RSZVL_VAL_ATV_STAN_K1", "Discrete or Min"=3.0, "Max"=0.0, "Coerced"=0.0, "Command"="K1"}, {"Name"="RSZVL_VAL_ATV_STAN_L", "Discrete or Min"=4.0, "Max"=0.0, "Coerced"=0.0, "Command"="L"}, {"Name"="RSZVL_VAL_ATV_STAN_M", "Discrete or Min"=5.0, "Max"=0.0, "Coerced"=0.0, "Command"="M"}, {"Name"="RSZVL_VAL_ATV_STAN_N", "Discrete or Min"=6.0, "Max"=0.0, "Coerced"=0.0, "Command"="N"}]}, {"Name"="rszvl_rngCatvDtvStandard", "Type"=2, "Min?"=FALSE, "Max?"=FALSE, "Entries"=[{"Name"="RSZVL_VAL_DTV_STAN_J83A", "Discrete or Min"=0.0, "Max"=0.0, "Coerced"=0.0, "Command"="J83A"}, {"Name"="RSZVL_VAL_DTV_STAN_J83B", "Discrete or Min"=1.0, "Max"=0.0, "Coerced"=0.0, "Command"="J83B"}, {"Name"="RSZVL_VAL_DTV_STAN_J83C", "Discrete or Min"=2.0, "Max"=0.0, "Coerced"=0.0, "Command"="J83C"}]}, {"Name"="rszvl_rngCatvAtvSoundSystem", "Type"=2, "Min?"=FALSE, "Max?"=FALSE, "Entries"=[{"Name"="RSZVL_VAL_ATV_AUDIO_FM55NICAM585", "Discrete or Min"=0.0, "Max"=0.0, "Coerced"=0.0, "Command"="FM55NICAM585"}, {"Name"="RSZVL_VAL_ATV_AUDIO_FM55FM5742", "Discrete or Min"=1.0, "Max"=0.0, "Coerced"=0.0, "Command"="FM55FM5742"}, {"Name"="RSZVL_VAL_ATV_AUDIO_FM55MONO", "Discrete or Min"=2.0, "Max"=0.0, "Coerced"=0.0, "Command"="FM55MONO"}, {"Name"="RSZVL_VAL_ATV_AUDIO_FM65NICAM585", "Discrete or Min"=3.0, "Max"=0.0, "Coerced"=0.0, "Command"="FM65NICAM585"}, {"Name"="RSZVL_VAL_ATV_AUDIO_FM65FM6258", "Discrete or Min"=4.0, "Max"=0.0, "Coerced"=0.0, "Command"="FM65FM6258"}, {"Name"="RSZVL_VAL_ATV_AUDIO_FM65FM6742", "Discrete or Min"=5.0, "Max"=0.0, "Coerced"=0.0, "Command"="FM65FM6742"}, {"Name"="RSZVL_VAL_ATV_AUDIO_FM65MONO", "Discrete or Min"=6.0, "Max"=0.0, "Coerced"=0.0, "Command"="FM65MONO"}, {"Name"="RSZVL_VAL_ATV_AUDIO_FM60NICAM6552", "Discrete or Min"=7.0, "Max"=0.0, "Coerced"=0.0, "Command"="FM60NICAM6552"}, {"Name"="RSZVL_VAL_ATV_AUDIO_FM60MONO", "Discrete or Min"=8.0, "Max"=0.0, "Coerced"=0.0, "Command"="FM60MONO"}, {"Name"="RSZVL_VAL_ATV_AUDIO_AM65NICAM585", "Discrete or Min"=9.0, "Max"=0.0, "Coerced"=0.0, "Command"="AM65NICAM585"}, {"Name"="RSZVL_VAL_ATV_AUDIO_AM60MONO", "Discrete or Min"=10.0, "Max"=0.0, "Coerced"=0.0, "Command"="AM60MONO"}, {"Name"="RSZVL_VAL_ATV_AUDIO_FM45BTSC", "Discrete or Min"=11.0, "Max"=0.0, "Coerced"=0.0, "Command"="FM45BTSC"}, {"Name"="RSZVL_VAL_ATV_AUDIO_FM45EIA_J", "Discrete or Min"=12.0, "Max"=0.0, "Coerced"=0.0, "Command"="FM45EIA_J"}, {"Name"="RSZVL_VAL_ATV_AUDIO_FM45FM4742", "Discrete or Min"=13.0, "Max"=0.0, "Coerced"=0.0, "Command"="FM45FM4742"}, {"Name"="RSZVL_VAL_ATV_AUDIO_FM45MONO", "Discrete or Min"=14.0, "Max"=0.0, "Coerced"=0.0, "Command"="FM45MONO"}]}, {"Name"="rszvl_rngCatvAtvColorSystem", "Type"=2, "Min?"=FALSE, "Max?"=FALSE, "Entries"=[{"Name"="RSZVL_VAL_ATV_COLOR_SYSTEM_PAL", "Discrete or Min"=0.0, "Max"=0.0, "Coerced"=0.0, "Command"="PAL"}, {"Name"="RSZVL_VAL_ATV_COLOR_SYSTEM_NTSC", "Discrete or Min"=1.0, "Max"=0.0, "Coerced"=0.0, "Command"="NTSC"}, {"Name"="RSZVL_VAL_ATV_COLOR_SYSTEM_SECAM", "Discrete or Min"=2.0, "Max"=0.0, "Coerced"=0.0, "Command"="SEC"}]}, {"Name"="rszvl_rngCatvDtvFormat", "Type"=2, "Min?"=FALSE, "Max?"=FALSE, "Entries"=[{"Name"="RSZVL_VAL_DTV_FORMAT_QAM4", "Discrete or Min"=0.0, "Max"=0.0, "Coerced"=0.0, "Command"="QAM4"}, {"Name"="RSZVL_VAL_DTV_FORMAT_QAM16", "Discrete or Min"=1.0, "Max"=0.0, "Coerced"=0.0, "Command"="QAM16"}, {"Name"="RSZVL_VAL_DTV_FORMAT_QAM32", "Discrete or Min"=2.0, "Max"=0.0, "Coerced"=0.0, "Command"="QAM32"}, {"Name"="RSZVL_VAL_DTV_FORMAT_QAM64", "Discrete or Min"=3.0, "Max"=0.0, "Coerced"=0.0, "Command"="QAM64"}, {"Name"="RSZVL_VAL_DTV_FORMAT_QAM128", "Discrete or Min"=4.0, "Max"=0.0, "Coerced"=0.0, "Command"="QAM128"}, {"Name"="RSZVL_VAL_DTV_FORMAT_QAM256", "Discrete or Min"=5.0, "Max"=0.0, "Coerced"=0.0, "Command"="QAM256"}, {"Name"="RSZVL_VAL_DTV_FORMAT_QAM512", "Discrete or Min"=6.0, "Max"=0.0, "Coerced"=0.0, "Command"="QAM512"}, {"Name"="RSZVL_VAL_DTV_FORMAT_QAM1024", "Discrete or Min"=7.0, "Max"=0.0, "Coerced"=0.0, "Command"="QAM1024"}]}, {"Name"="rszvl_rngCatvAtvTriggField", "Type"=0, "Min?"=TRUE, "Max?"=TRUE, "Entries"=[{"Name"="", "Discrete or Min"=1.0, "Max"=2.0, "Coerced"=0.0, "Command"=""}]}, {"Name"="rszvl_rngCatvAtvTriggBarLineType", "Type"=2, "Min?"=FALSE, "Max?"=FALSE, "Entries"=[{"Name"="RSZVL_VAL_ATV_BLIN_TYPE_CCIR17", "Discrete or Min"=0.0, "Max"=0.0, "Coerced"=0.0, "Command"="CCIR17"}, {"Name"="RSZVL_VAL_ATV_BLIN_TYPE_FCC", "Discrete or Min"=1.0, "Max"=0.0, "Coerced"=0.0, "Command"="FCC"}, {"Name"="RSZVL_VAL_ATV_BLIN_TYPE_NTC7", "Discrete or Min"=2.0, "Max"=0.0, "Coerced"=0.0, "Command"="NTC7"}]}, {"Name"="rszvl_rngCatvPowerUnits", "Type"=2, "Min?"=FALSE, "Max?"=FALSE, "Entries"=[{"Name"="RSZVL_VAL_UNIT_DBM", "Discrete or Min"=0.0, "Max"=0.0, "Coerced"=0.0, "Command"="DBM"}, {"Name"="RSZVL_VAL_UNIT_DBPW", "Discrete or Min"=1.0, "Max"=0.0, "Coerced"=0.0, "Command"="DBPW"}, {"Name"="RSZVL_VAL_UNIT_WATT", "Discrete or Min"=2.0, "Max"=0.0, "Coerced"=0.0, "Command"="W"}, {"Name"="RSZVL_VAL_UNIT_DBUV", "Discrete or Min"=3.0, "Max"=0.0, "Coerced"=0.0, "Command"="DBUV"}, {"Name"="RSZVL_VAL_UNIT_DBMV", "Discrete or Min"=4.0, "Max"=0.0, "Coerced"=0.0, "Command"="DBMV"}, {"Name"="RSZVL_VAL_UNIT_VOLT", "Discrete or Min"=5.0, "Max"=0.0, "Coerced"=0.0, "Command"="V"}, {"Name"="RSZVL_VAL_UNIT_DBUA", "Discrete or Min"=6.0, "Max"=0.0, "Coerced"=0.0, "Command"="DBUA"}, {"Name"="RSZVL_VAL_UNIT_AMP", "Discrete or Min"=7.0, "Max"=0.0, "Coerced"=0.0, "Command"="A"}]}, {"Name"="rszvl_rngCatvResults", "Type"=2, "Min?"=FALSE, "Max?"=FALSE, "Entries"=[{"Name"="RSZVL_VAL_RES_FAIL", "Discrete or Min"=0.0, "Max"=0.0, "Coerced"=0.0, "Command"="FAIL"}, {"Name"="RSZVL_VAL_RES_PASS", "Discrete or Min"=1.0, "Max"=0.0, "Coerced"=0.0, "Command"="PASS"}]}, {"Name"="rszvl_rngPmetMeasTime", "Type"=2, "Min?"=FALSE, "Max?"=FALSE, "Entries"=[{"Name"="RSZVL_VAL_PMET_MEASTIME_NORM", "Discrete or Min"=0.0, "Max"=0.0, "Coerced"=0.0, "Command"="NORM"}, {"Name"="RSZVL_VAL_PMET_MEASTIME_SHORT", "Discrete or Min"=1.0, "Max"=0.0, "Coerced"=0.0, "Command"="SHOR"}, {"Name"="RSZVL_VAL_PMET_MEASTIME_LONG", "Discrete or Min"=2.0, "Max"=0.0, "Coerced"=0.0, "Command"="LONG"}]}, {"Name"="rszvl_rngPmetCoupling", "Type"=2, "Min?"=FALSE, "Max?"=FALSE, "Entries"=[{"Name"="RSZVL_VAL_PMET_COUP_OFF", "Discrete or Min"=0.0, "Max"=0.0, "Coerced"=0.0, "Command"="OFF"}, {"Name"="RSZVL_VAL_PMET_COUP_CENT", "Discrete or Min"=1.0, "Max"=0.0, "Coerced"=0.0, "Command"="CENT"}, {"Name"="RSZVL_VAL_PMET_COUP_MARK", "Discrete or Min"=2.0, "Max"=0.0, "Coerced"=0.0, "Command"="MARK"}]}, {"Name"="rszvl_rngPmetUnitAbs", "Type"=2, "Min?"=FALSE, "Max?"=FALSE, "Entries"=[{"Name"="RSZVL_VAL_UNIT_DBM", "Discrete or Min"=0.0, "Max"=0.0, "Coerced"=0.0, "Command"="DBM"}, {"Name"="RSZVL_VAL_UNIT_WATT", "Discrete or Min"=2.0, "Max"=0.0, "Coerced"=0.0, "Command"="WATT"}]}, {"Name"="rszvl_rngPmetUnitRel", "Type"=2, "Min?"=FALSE, "Max?"=FALSE, "Entries"=[{"Name"="RSZVL_VAL_UNIT_DB", "Discrete or Min"=8.0, "Max"=0.0, "Coerced"=0.0, "Command"="DB"}, {"Name"="RSZVL_VAL_UNIT_PCT", "Discrete or Min"=13.0, "Max"=0.0, "Coerced"=0.0, "Command"="PCT"}]}, {"Name"="rszvl_rngUnitLength", "Type"=2, "Min?"=FALSE, "Max?"=FALSE, "Entries"=[{"Name"="RSZVL_VAL_UNIT_LEN_METER", "Discrete or Min"=0.0, "Max"=0.0, "Coerced"=0.0, "Command"="MET"}, {"Name"="RSZVL_VAL_UNIT_LEN_FOOT", "Discrete or Min"=1.0, "Max"=0.0, "Coerced"=0.0, "Command"="FOOT"}]}, {"Name"="rszvl_rngRipplePhysicalUnits", "Type"=2, "Min?"=FALSE, "Max?"=FALSE, "Entries"=[{"Name"="RSZVL_VAL_RIPP_PHYS_UNIT_FLIN", "Discrete or Min"=0.0, "Max"=0.0, "Coerced"=0.0, "Command"="FLIN"}, {"Name"="RSZVL_VAL_RIPP_PHYS_UNIT_FLOG", "Discrete or Min"=1.0, "Max"=0.0, "Coerced"=0.0, "Command"="FLOG"}, {"Name"="RSZVL_VAL_RIPP_PHYS_UNIT_FSEG", "Discrete or Min"=2.0, "Max"=0.0, "Coerced"=0.0, "Command"="FSEG"}, {"Name"="RSZVL_VAL_RIPP_PHYS_UNIT_FSIN", "Discrete or Min"=3.0, "Max"=0.0, "Coerced"=0.0, "Command"="FSIN"}, {"Name"="RSZVL_VAL_RIPP_PHYS_UNIT_TLIN", "Discrete or Min"=4.0, "Max"=0.0, "Coerced"=0.0, "Command"="TLIN"}, {"Name"="RSZVL_VAL_RIPP_PHYS_UNIT_TLOG", "Discrete or Min"=5.0, "Max"=0.0, "Coerced"=0.0, "Command"="TLOG"}, {"Name"="RSZVL_VAL_RIPP_PHYS_UNIT_PLIN", "Discrete or Min"=6.0, "Max"=0.0, "Coerced"=0.0, "Command"="PLIN"}, {"Name"="RSZVL_VAL_RIPP_PHYS_UNIT_PLOG", "Discrete or Min"=7.0, "Max"=0.0, "Coerced"=0.0, "Command"="PLOG"}, {"Name"="RSZVL_VAL_RIPP_PHYS_UNIT_PSIN", "Discrete or Min"=8.0, "Max"=0.0, "Coerced"=0.0, "Command"="PSIN"}]}, {"Name"="rszvl_rngRippleFormUnits", "Type"=2, "Min?"=FALSE, "Max?"=FALSE, "Entries"=[{"Name"="RSZVL_VAL_RIPP_FORM_UNIT_COMP", "Discrete or Min"=0.0, "Max"=0.0, "Coerced"=0.0, "Command"="COMP"}, {"Name"="RSZVL_VAL_RIPP_FORM_UNIT_MAGN", "Discrete or Min"=1.0, "Max"=0.0, "Coerced"=0.0, "Command"="MAGN"}, {"Name"="RSZVL_VAL_RIPP_FORM_UNIT_PHAS", "Discrete or Min"=2.0, "Max"=0.0, "Coerced"=0.0, "Command"="PHAS"}, {"Name"="RSZVL_VAL_RIPP_FORM_UNIT_REAL", "Discrete or Min"=3.0, "Max"=0.0, "Coerced"=0.0, "Command"="REAL"}, {"Name"="RSZVL_VAL_RIPP_FORM_UNIT_IMAG", "Discrete or Min"=4.0, "Max"=0.0, "Coerced"=0.0, "Command"="IMAG"}, {"Name"="RSZVL_VAL_RIPP_FORM_UNIT_SWR", "Discrete or Min"=5.0, "Max"=0.0, "Coerced"=0.0, "Command"="SWR"}, {"Name"="RSZVL_VAL_RIPP_FORM_UNIT_GDEL", "Discrete or Min"=6.0, "Max"=0.0, "Coerced"=0.0, "Command"="GDEL"}, {"Name"="RSZVL_VAL_RIPP_FORM_UNIT_L", "Discrete or Min"=7.0, "Max"=0.0, "Coerced"=0.0, "Command"="L"}, {"Name"="RSZVL_VAL_RIPP_FORM_UNIT_C", "Discrete or Min"=8.0, "Max"=0.0, "Coerced"=0.0, "Command"="C"}]}, {"Name"="rszvl_rngTraceAperture", "Type"=0, "Min?"=TRUE, "Max?"=TRUE, "Entries"=[{"Name"="", "Discrete or Min"=1.0, "Max"=10000.0, "Coerced"=0.0, "Command"=""}]}, {"Name"="rszvl_rngEventStart", "Type"=2, "Min?"=FALSE, "Max?"=FALSE, "Entries"=[{"Name"="RSZVL_VAL_TRG_START_SWEEP", "Discrete or Min"=0.0, "Max"=0.0, "Coerced"=0.0, "Command"="'SWE'"}, {"Name"="RSZVL_VAL_TRG_START_POINT", "Discrete or Min"=1.0, "Max"=0.0, "Coerced"=0.0, "Command"="'POIN'"}]}] {"Type" items=["Range", "Coerced", "Discrete"]}
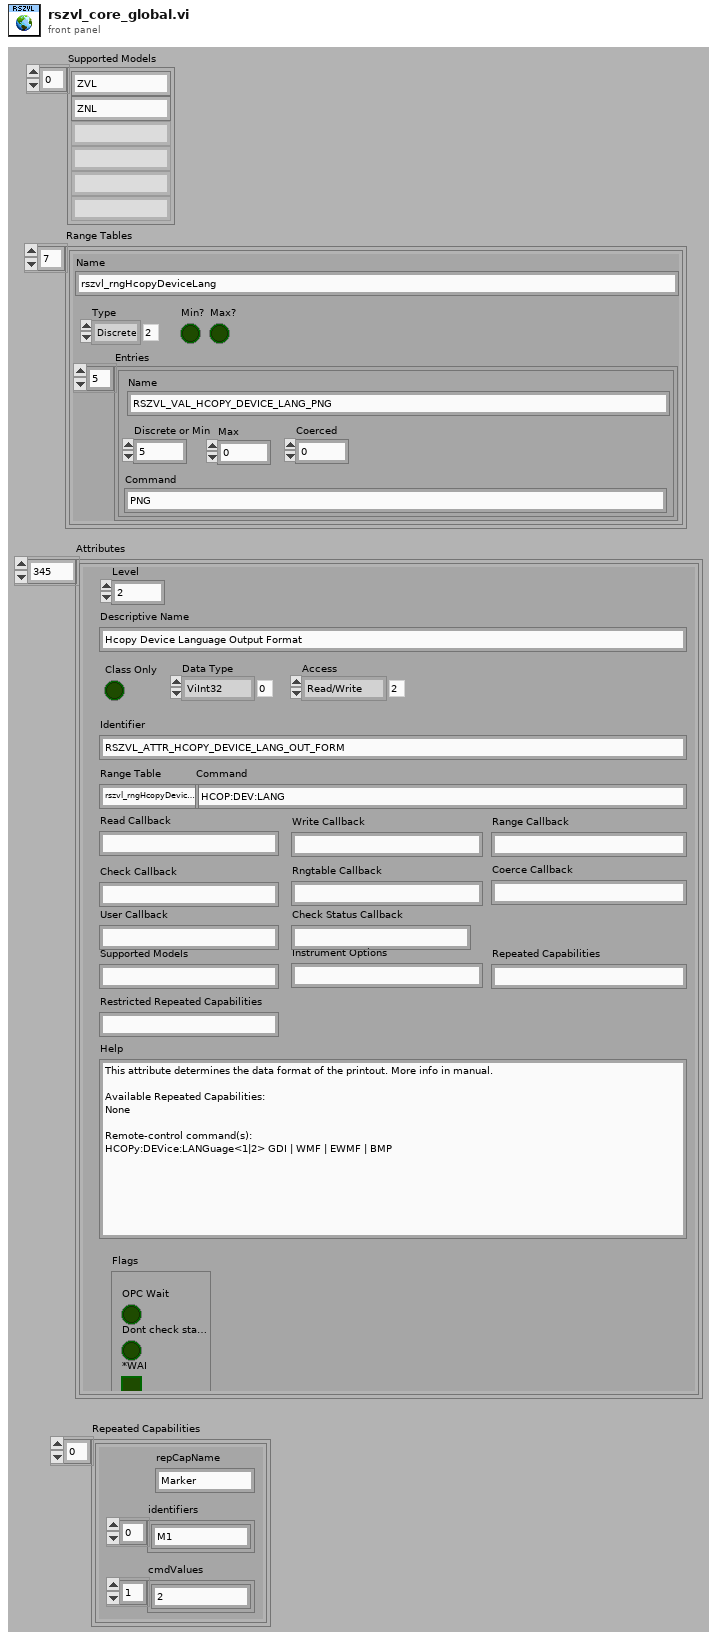
[diagram p1: front panel]
types:
  T1 = cluster{"repCapName":string, "identifiers":string[], "cmdValues":string[]}[]
  T2 = cluster{"Level":i32, "Descriptive Name":string, "Class Only":bool, "Data Type":u16, "Access":u16, "Identifier":string, "Range Table":string, "Command":string, "Read Callback":string, "Write Callback":string, "Range Callback":string, "Check Callback":string, "Rngtable Callback":string, "Coerce Callback":string, "User Callback":string, "Supported Models":string, "Instrument Options":string, "Repeated Capabilities":string, "Restricted Repeated Capabilities":string, "Help":string, "Flags":cluster{"OPC Wait":bool, "Dont check status":bool, "*WAI":bool}, "Check Status Callback":string}[]
  T3 = cluster{"Name":string, "Type":i32, "Min?":bool, "Max?":bool, "Entries":cluster{"Name":string, "Discrete or Min":dbl, "Max":dbl, "Coerced":dbl, "Command":string}[]}[]
diagram:
